vi "Read refs_controls_V0_VD2.vi"(8 "error in (no error)":errorcluster, 10 "EXP":bool=TRUE caption="EXP V0/VD2", 11 "Control-Client in":refnum<class "Control-Client.lvclass">) -> (0 "error out":errorcluster, 2 "refs_controls":refnum<vi>[](array[refnum]), 3 "Control-Client out":refnum<class "Control-Client.lvclass">)   [LabVIEW 2019, in "Control-Client.lvclass"]
uses:
  Control-Client.lvclass
  Control-Client.lvclass/Control-Client.ctl
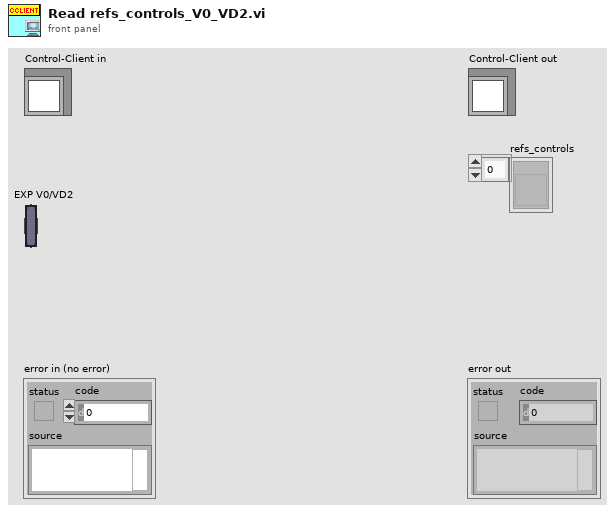
[diagram p1: front panel]
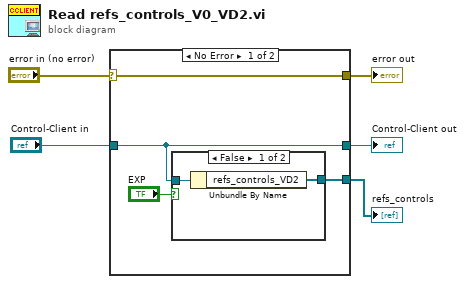
[diagram p0: block diagram]
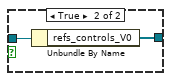
[diagram p2: hidden frame]
diagram:
  n1 = case shown="No Error" "error in (no error)" {
    selector: "error in (no error)" -> [w9 w14]
    tunnel: [w9 w14] -> w4
    tunnel: [w7 w15] -> w2
    tunnel: "Control-Client in" -> [w7 w15]
    tunnel: [w6 _] -> w1
    frame No Error {
      n2 = case shown="False" "EXP" {
        tunnel: w7 -> [w11 w12]
        tunnel: [w10 w13] -> w6
        frame False {
          n3 = Unbundle By Name(w11) -> ("refs_controls_VD2"=w10:refnum<vi>[])
        }
        frame True {
          n4 = Unbundle By Name(w12) -> ("refs_controls_V0"=w13:refnum<vi>[])
        }
      }
    }
    frame Error {
    }
  }
  "error out" <- w4
  "Control-Client out" <- w2
  "refs_controls" <- w1
